vi "Teardown.vi"(8 "error in (no error)":errorcluster, 11 "Teardown Error In":refnum<class "Teardown Error.lvclass">) -> (0 "error out":errorcluster, 3 "Teardown Error Out":refnum<class "Teardown Error.lvclass">)   [LabVIEW 2020, in "Teardown Error.lvclass"]
doc: "Teardown method called by the testing framework to tear down test fixture after each test method is called."
uses:
  Teardown Error.lvclass
  source/LUnit Test Case.lvclass
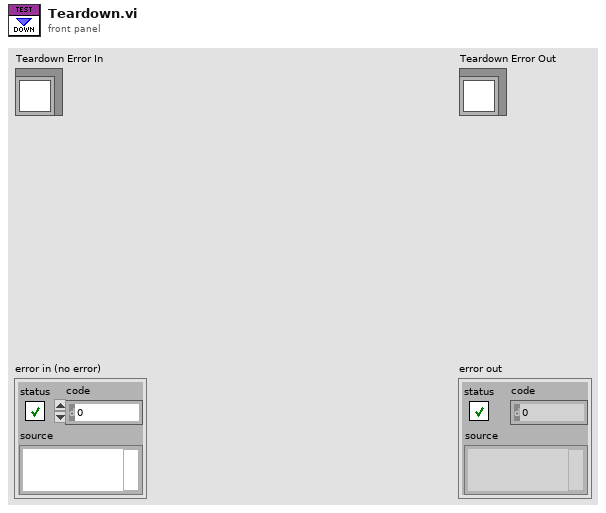
[diagram p1: front panel]
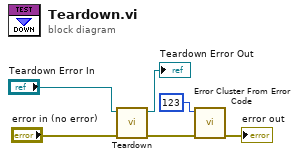
[diagram p0: block diagram]
diagram:
  n1 = call-parent "Teardown.vi"("error in (no error)"="error in (no error)", "LUnit Test Case In"="Teardown Error In") -> ("error out"=w6:errorcluster, "LUnit Test Case Out"=→"Teardown Error Out":refnum<class "Teardown Error.lvclass">)  [unwired: 8 in]
  n2 = call <vilib>:"Error Cluster From Error Code.vi"("error in (no error)"=w6, "error code (0)"=123) -> ("error out"=→"error out":errorcluster)  [unwired: 7 in]
